vi "Get RFM Interrupt Enabled States.vi"(8 "error in (no error)":errorcluster, 11 "GE 5565PIORC in":refnum<class "GE 5565PIORC.lvclass">) -> (0 "error out":errorcluster, 2 "Interrupt Enables":T1, 3 "GE 5565PIORC out":refnum<class "GE 5565PIORC.lvclass">)   [LabVIEW 2016, in "GE 5565PIORC.lvclass"]
uses:
  GE 5565PIORC.lvclass
  Controls/Interrupt Enables.ctl
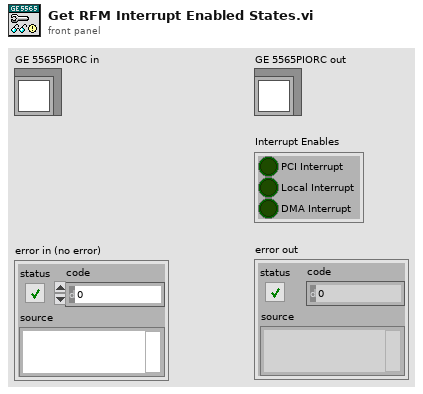
[diagram p1: front panel]
types:
  T1 = typedef "GE 5565PIORC.lvclass/Interrupt Enables.ctl" = cluster{"PCI Interrupt":bool, "Local Interrupt":bool, "DMA Interrupt":bool}
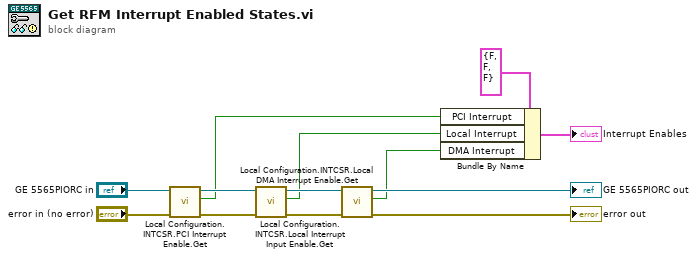
[diagram p0: block diagram]
diagram:
  n1 = call "Local Configuration.INTCSR.PCI Interrupt Enable.Get.vi"("error in (no error)"="error in (no error)", "GE 5565PIORC"="GE 5565PIORC in") -> ("error out"=w8:errorcluster, "PCI Interrupt Enabled?"=w3:bool, "GE 5565PIORC out"=w9:refnum<class "GE 5565PIORC.lvclass">)  [unwired: 7 in]
  n2 = call "Local Configuration.INTCSR.Local Interrupt Input Enable.Get.vi"("error in (no error)"=w8, "GE 5565PIORC"=w9) -> ("error out"=w6:errorcluster, "Local Interrupt Input Enabled?"=w2:bool, "GE 5565PIORC out"=w7:refnum<class "GE 5565PIORC.lvclass">)  [unwired: 7 in]
  n3 = call "Local Configuration.INTCSR.Local DMA Interrupt Enable.Get.vi"("error in (no error)"=w6, "GE 5565PIORC"=w7) -> ("error out"=→"error out":errorcluster, "Local DMA Interrupt Enabled?"=w1:bool, "GE 5565PIORC out"=→"GE 5565PIORC out":refnum<class "GE 5565PIORC.lvclass">)  [unwired: 7 in]
  n4 = Bundle By Name(cluster=T1 {"PCI Interrupt"=FALSE, "Local Interrupt"=FALSE, "DMA Interrupt"=FALSE} ("Interrupt Enables"), "PCI Interrupt"=w3, "Local Interrupt"=w2, "DMA Interrupt"=w1) -> (→"Interrupt Enables":T1)
